vi "Read CPU IP Address.vi"(8 "error in (no error)":errorcluster, 11 "base path":path) -> (0 "error out":errorcluster, 2 "IP Address":string[](array[string]), 3 "configuration file path out":path)   [LabVIEW 2014]
uses:
  Operation File/ini/type defs/ini file actions.ctl
  <vilib>/Utility/config.llb/NI_LVConfig.lvlib
  Operation File/ini/type defs/ini entry value.ctl
  Operation File/ini/type defs/ini entry types.ctl
  Operation File/ini/type defs/ini entry.ctl
  Simatic S7.lvlib
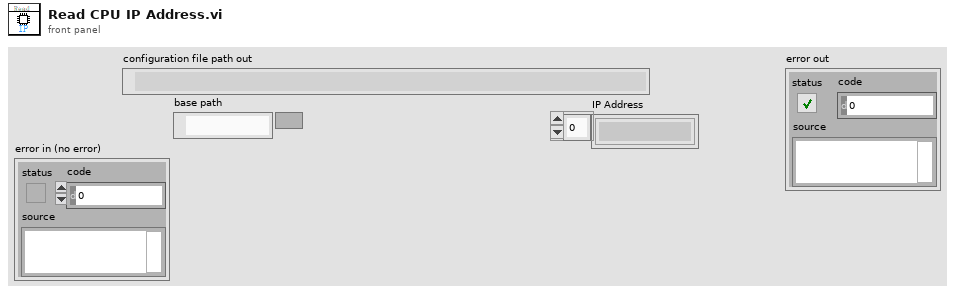
[diagram p1: front panel]
types:
  T1 = typedef "ini entry.ctl" = cluster{"section":string, "key":string, "type":T2, "default value":T3}
  T2 = typedef "ini entry types.ctl" = enum16{"Boolean", "Double", "I32", "Path", "String", "U32"}
  T3 = typedef "ini entry value.ctl" = cluster{"Boolean":bool, "Dbl":dbl, "I32":i32, "Path":path, "String":string, "U32":u32}
  T4 = typedef "Simatic S7.lvlib/Op ip address.ctl" = enum16{"Init", "Add IP", "Get IP"}
  T5 = typedef "Simatic S7.lvlib/Siemens Ref.ctl" = cluster{"IP Address ":string, "Conn ID":refnum<k5>, "Timeout ms":i32, "Status":bool, "Slot":u16, "Rack":u16}
  T6 = typedef "ini file actions.ctl" = enum16{"read ini", "write ini"}
  T7 = typedef "NI_LVConfig.lvlib/Config Data RefNum.ctl" = refnum<k1>
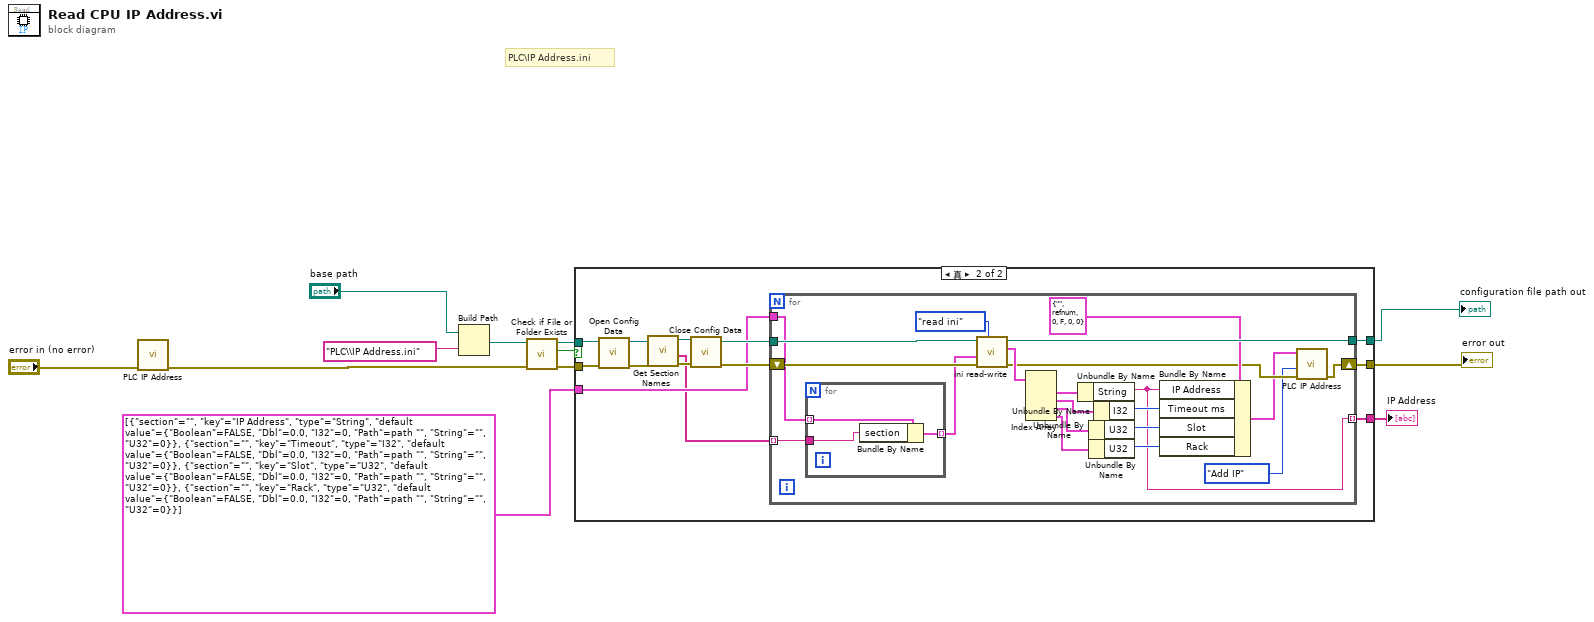
[diagram p0: block diagram]
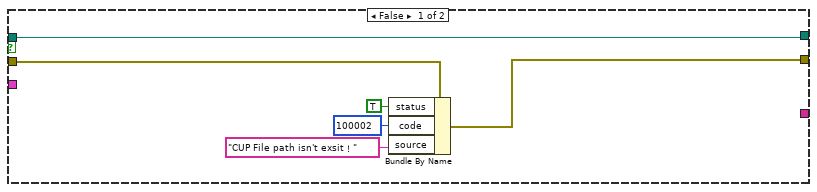
[diagram p2: hidden frame]
diagram:
  # "PLC\\IP Address.ini"
  n1 = call "PLC IP Address.vi"("error in (no error)"="error in (no error)") -> ("error out"=w3:errorcluster)  [unwired: 8 in, 2 out]
  n2 = Build Path(base path="base path", name or relative path="PLC\\IP Address.ini") -> (appended path=w11:path)
  n3 = call <vilib>:"Check if File or Folder Exists.vi"("error in (no error)"=w3, "path"=w11) -> ("error out"=w9:errorcluster, "file or folder exists?"=w10:bool, "dup path"=w8:path)  [unwired: 7 in]
  n4 = case shown="真" w10 {
    tunnel: w9 -> [w17 w31]
    tunnel: w8 -> [w18 w30]
    tunnel: T1[] [{"section"="", "key"="IP Address", "type"=enum."String", "default value"={"Boolean"=FALSE, "Dbl"=0.0, "I32"=0, "Path"=path "", "String"="", "U32"=0}}, {"section"="", "key"="Timeout", "type"=enum."I32", "default value"={"Boolean"=FALSE, "Dbl"=0.0, "I32"=0, "Path"=path "", "String"="", "U32"=0}}, {"section"="", "key"="Slot", "type"=enum."U32", "default value"={"Boolean"=FALSE, "Dbl"=0.0, "I32"=0, "Path"=path "", "String"="", "U32"=0}}, {"section"="", "key"="Rack", "type"=enum."U32", "default value"={"Boolean"=FALSE, "Dbl"=0.0, "I32"=0, "Path"=path "", "String"="", "U32"=0}}] ("ini entry descriptors") -> [_ w23]
    tunnel: [w18 w21] -> w5
    tunnel: [w16 w20] -> w6
    tunnel: [_ w19] -> w1
    frame False {
      n5 = Bundle By Name(cluster=w17, "status"=TRUE, "code"=100002, "source"="CUP File path isn't exsit！") -> (w16:errorcluster)
    }
    frame True {
      n6 = call <vilib>:"Open Config Data.vi"("error in (no error)"=w31, "configuration file path"=w30) -> ("error out"=w29:errorcluster, "refnum"=w28:T7)  [unwired: 7 in, 1 out]
      n7 = call <vilib>:"Get Section Names.vi"("error in (no error)"=w29, "refnum"=w28) -> ("error out"=w27:errorcluster, "section names"=w22:string[], "refnum out"=w26:T7)  [unwired: 7 in]
      n8 = call <vilib>:"Close Config Data.vi"("error in (no error)"=w27, "refnum"=w26) -> ("error out"=w25:errorcluster, "file path"=w24:path)  [unwired: 8 in]
      n9 = for {
        tunnel: w24 -> [w50]
        tunnel: w23 -> [w49]
        tunnel: w22 -> [w48] mode=indexing
        shift-right: [w35] -> w20
        shift-left: w25 -> [w51]
        tunnel: [w41] -> w21
        tunnel: [w32] -> w19 mode=indexing
        n10 = for {
          tunnel: w49 -> [w55] mode=indexing
          tunnel: w48 -> [w54]
          tunnel: [w53] -> w47 mode=indexing
          n11 = Bundle By Name(cluster=w55, "section"=w54) -> (w53:T1)
        }
        n12 = call "ini read-write.vi"("action"=ini_file_actions."read ini", "error in (no error)"=w51, "ini entry descriptors"=w47, "configuration file path"=w50) -> ("error out"=w36:errorcluster, "values out"=w46:T3[], "configuration file path out"=w41:path)  [unwired: 5 in]
        n13 = Index Array(array=w46) -> (element #1=w45:T3, element #2=w44:T3, element #3=w43:T3, element #4=w42:T3)  [unwired: 4 in]
        n14 = Unbundle By Name(w45) -> ("String"=w32:string)
        n15 = Unbundle By Name(w43) -> ("U32"=w38:u32)
        n16 = Unbundle By Name(w42) -> ("U32"=w37:u32)
        n17 = Unbundle By Name(w44) -> ("I32"=w39:i32)
        n18 = Bundle By Name(cluster=T5 {"IP Address "="", "Conn ID"=refnum, "Timeout ms"=0, "Status"=FALSE, "Slot"=0, "Rack"=0} ("Siemens Ctr"), "IP Address"=w32, "Timeout ms"=w39, "Slot"=w38, "Rack"=w37) -> (w33:T5)
        n19 = call "PLC IP Address.vi"("error in (no error)"=w36, "Operationip"=Op_ip_address."Add IP", "Siemens Ctr"=w33) -> ("error out"=w35:errorcluster)  [unwired: 6 in, 2 out]
      }
    }
  }
  "error out" <- w6
  "configuration file path out" <- w5
  "IP Address" <- w1
